vi "DAQmx Create Channel (AO-Voltage-Basic).vi"(0 "task in":refnum<k21>, 1 "maximum value":dbl=10.0 format="%0.2f", 2 "minimum value":dbl=-10.0 format="%0.2f", 3 "output terminal configuration":i32(ring)=-1 items=["Default"=-1, "RSE"=10083, "Differential"=10106, "Pseudodifferential"=12529], 5 "physical channels":tag, 7 "name to assign":string, 9 "units":i32(ring)=10348 items=["Volts"=10348, "From Custom Scale"=10065], 11 "error in":errorcluster, 12 "custom scale name":tag) -> (4 "task out":refnum<k21>, 15 "error out":errorcluster)   [LabVIEW 2011]
doc: "Creates channel(s) to generate voltage."
uses:
  C:/Program Files/National Instruments/LabVIEW 2011/resource/objmgr/daqmx.rc
panel:
  # "output limits"
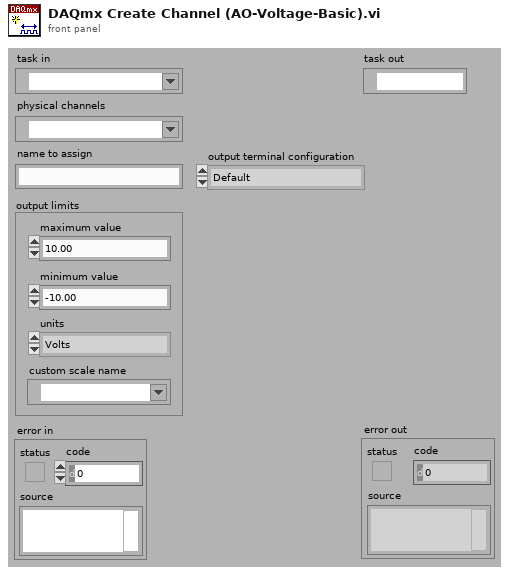
[diagram p1: front panel]
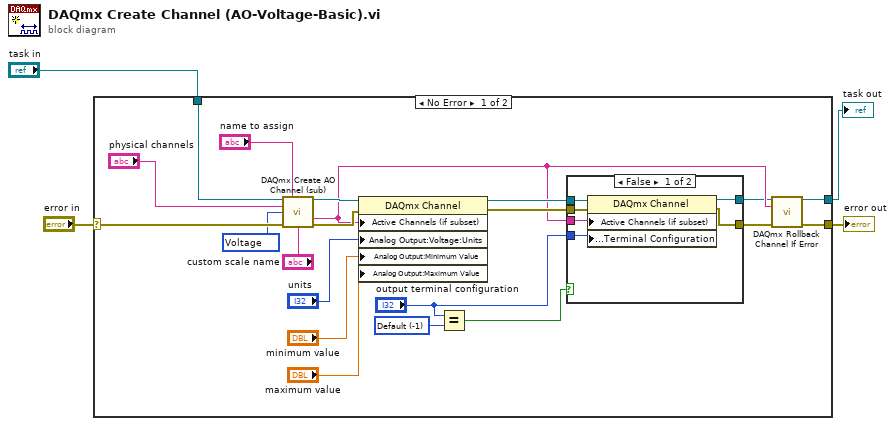
[diagram p0: block diagram]
diagram:
  n1 = case shown="No Error" "error in" {
    selector: "error in" -> [w24 w35]
    tunnel: [w14 w35] -> w4
    tunnel: "task in" -> [w25 w34]
    tunnel: [w13 w34] -> w1
    frame No Error {
      w12 = -1 items=["Default"=-1, "Differential"=10106, "Pseudodifferential"=12529] ("output terminal configuration")
      w17 = 10322 items=["Voltage"=10322, "Current"=10134] ("output type")
      n2 = call "DAQmx Create AO Channel (sub).vi"("task in"=w25, "virtual channel name"="name to assign", "physical channel name"="physical channels", "output type"=w17, "error in"=w24, "custom scale"="custom scale name") -> ("task out"=w15:refnum<k21>, "channel names"=w8:string, "error out"=w22:errorcluster)  [unwired: 7 out]
      n3 = property class="DAQmx Channel"(reference=w15, error in=w22, "Active Channels (if subset)"=w8, "Analog Output:Voltage:Units"="units", "Analog Output:Minimum Value"="minimum value", "Analog Output:Maximum Value"="maximum value") -> (reference out=w10:refnum<k21>, error out=w9:errorcluster)
      n4 = Equal?(x="output terminal configuration", y=w12) -> (x = y?=w11:bool)
      n5 = case shown="False" w11 {
        tunnel: w10 -> [w31 w33]
        tunnel: w9 -> [w30 w32]
        tunnel: w8 -> [w29 _]
        tunnel: "output terminal configuration" -> [w28 _]
        tunnel: [w27 w33] -> w6
        tunnel: [w26 w32] -> w5
        frame False {
          n6 = property class="DAQmx Channel"(reference=w31, error in=w30, "Active Channels (if subset)"=w29, "Analog Output:General Properties:Output Configuration:Terminal Configuration"=w28) -> (reference out=w27:refnum<k21>, error out=w26:errorcluster)
        }
        frame True {
        }
      }
      n7 = call "DAQmx Rollback Channel If Error.vi"("task in"=w6, "channel names"=w8, "error in"=w5) -> ("task out"=w13:refnum<k21>, "error out"=w14:errorcluster)  [unwired: 11 out]
    }
    frame Error {
    }
  }
  "error out" <- w4
  "task out" <- w1
